vi "PID.vi"() -> ()   [LabVIEW 2019]
panel:
  in  "TURNING":cluster{"P":dbl, "I":dbl, "D":dbl}
  in  "SHOOTER ANGLE":T1
  in  "CLIMBER ARM":T1
  in  "INTAKE PIVOT":T1
  in  "SHOOTER":T1
  in  "TURRET":T1
  in  "MOTION PROFILE":T1
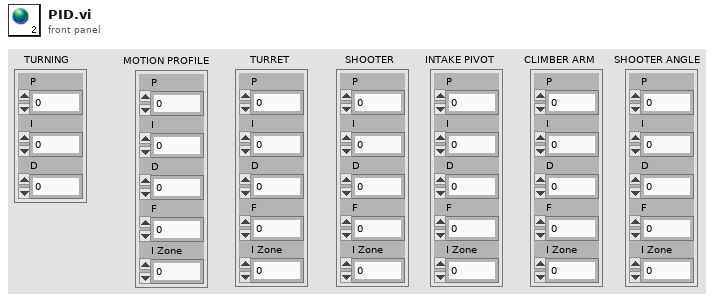
[diagram p1: front panel]
types:
  T1 = cluster{"P":dbl, "I":dbl, "D":dbl, "F":dbl, "I Zone":dbl}
diagram:
